vi "DFD Probe Check Filter Bank.vi"(1 "filter bank in":T1={"mFBank_AnalysisFilters"=[], "mFBank_SynthesisFilters"=[], "mFBank_#Bands"=0, "mFBank_ProcMethod"=enum."General", "mFBank_Coeffs"=[], "mFBank_Gain"=1.0, "mFBank_Delay"=0, "mFBank_Type"=0} {"mFBank_SynthesisFilters"."mMRate_SumWl" min=1 max=32 step=1; "mFBank_SynthesisFilters"."mMRate_InputIwl" min=1 max=32 step=1; "mFBank_SynthesisFilters"."mMRate_GainWl" min=1 max=32 step=1; "mFBank_SynthesisFilters"."mMRate_OutputWl" min=1 max=32 step=1; "mFBank_SynthesisFilters"."mMRate_InputWl" min=1 max=32 step=1; "mFBank_SynthesisFilters"."mMRate_CoefWl" min=1 max=32 step=1; "mFBank_SynthesisFilters"."mMRate_Mode" items=["Default"=-1, "No Rate Change"=0, "Interpolation"=1, "Decimation"=2, "Interpolated"=3, "Rational"=4]; "mFBank_AnalysisFilters"."mMRate_SumWl" min=1 max=32 step=1; "mFBank_AnalysisFilters"."mMRate_InputIwl" min=1 max=32 step=1; "mFBank_AnalysisFilters"."mMRate_GainWl" min=1 max=32 step=1; "mFBank_AnalysisFilters"."mMRate_OutputWl" min=1 max=32 step=1; "mFBank_AnalysisFilters"."mMRate_InputWl" min=1 max=32 step=1; "mFBank_AnalysisFilters"."mMRate_CoefWl" min=1 max=32 step=1; "mFBank_AnalysisFilters"."mMRate_Mode" items=["Default"=-1, "No Rate Change"=0, "Interpolation"=1, "Decimation"=2, "Interpolated"=3, "Rational"=4]; "mFBank_Type" items=["Uniform", "Non-Uniform"]}) -> (0 "Boolean":bool)   [LabVIEW 2017, in "NI_DigFilterLicensed.lvlib"]
uses:
  <vilib>/addons/Digital Filter Design/NI_DigFilterLicensed.lvlib
  <vilib>/addons/Digital Filter Design/FilterBank.llb/Object/DFD Filter Bank Obj.ctl
  <vilib>/addons/Digital Filter Design/_Objects.llb/DFD Multirate Filter Obj.ctl
  <vilib>/addons/Digital Filter Design/_Objects.llb/DFD Multirate Mode.ctl
  <vilib>/addons/Digital Filter Design/_Objects.llb/DFD Coef Norm Type.ctl
  <vilib>/addons/Digital Filter Design/_Objects.llb/DFD Round-off Mode.ctl
  <vilib>/addons/Digital Filter Design/_Objects.llb/DFD FXP MRate Multiply Mode.ctl
  <vilib>/addons/Digital Filter Design/FilterBank.llb/Object/DFD Filter Bank Processing Method.ctl
  <vilib>/addons/Digital Filter Design/FilterBank.llb/Object/DFD Filter Bank Type.ctl
  <vilib>/addons/Digital Filter Design/NI_DigFilter_FilterBank.lvlib
panel:
  in  "Tab Control":T9(tab)
  in  "order":i32=-1 caption="Filter bank order" min=2
  in  "#bands":i32 caption="Number of bands" min=1 max=1 step=1
  in  "dist_in dB":bool=TRUE caption="Magnitude in dB"
  out "Mag distortion":cluster{dbl[], "values":dbl[]}(graph)
  in  "resp_in dB":bool=TRUE caption="Magnitude in dB"
  out "Mag responses":cluster{"Y":dbl[], "Y":dbl[]}[](graph)
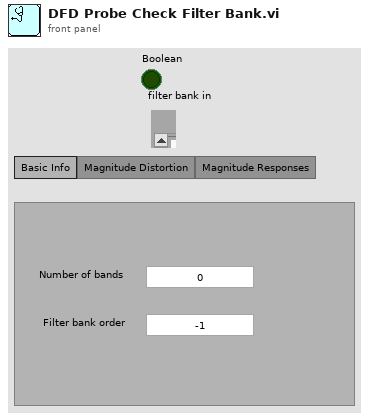
[diagram p1: front panel]
types:
  T1 = typedef "NI_DigFilter_FilterBank.lvlib/DFD Filter Bank Obj.ctl" = cluster{"mFBank_AnalysisFilters":T2[], "mFBank_SynthesisFilters":T2[], "mFBank_#Bands":i32, "mFBank_ProcMethod":T7, "mFBank_Coeffs":dbl[], "mFBank_Gain":dbl, "mFBank_Delay":i32, "mFBank_Type":T8}
  T2 = typedef "NI_DigFilterLicensed.lvlib/DFD Multirate Filter Obj.ctl" = cluster{"mMRate_Structure":enum16{"CIC", "FIR", "IIR", "Lattice"}, "mMRate_Mode":T3, "mMRate_Factor":i32, "mMRate_FIRParams":cluster{"mMRate_FIR_H":dbl[], "mMRate_FIR_IsNyquist?":bool, "mMRate_FIR_IsSymmetric?":bool}, "mMRate_CICParams":cluster{"mMRate_CIC_#Stage":i32, "mMRate_CIC_Lag":i32, "mMRate_CIC_Type":enum16{"Lowpass", "Highpass"}}, "mMRate_Order":i32, "mMRate_Version":string, "mMRate_Comments":string, "mMRate_RationalFactor":cluster{"mMRate_L":i32, "mMRate_M":i32}, "mMRate_Fs":dbl, "mMRate_Quantized?":bool, "mMRate_QFilterGain":dbl, "mMRate_CoefWl":i16, "mMRate_Scaling":cluster{"mMRate_ScaleByPowerOf2?":bool, "mMRate_ScaleType":T4}, "mMRate_InputWl":i16, "mMRate_OutputWl":i16, "mMRate_OutputMode":T5, "mMRate_MultMode":T6, "mMRate_BitPruning":bool, "mMRate_GainWl":i16, "mMRate_OutputFwl":i16, "mMRate_SumIwl":i16, "mMRate_InputIwl ":i16, "mMRate_SumWl":i16, "mMRate_CoefIwl":i16}
  T3 = typedef "NI_DigFilterLicensed.lvlib/DFD Multirate Mode.ctl" = i16
  T4 = typedef "NI_DigFilterLicensed.lvlib/DFD Coef Norm Type.ctl" = enum16{"No Norm", "Time Domain 1-Norm", "Time Domain 2-Norm", "Time Domain Inf-Norm"}
  T5 = typedef "NI_DigFilterLicensed.lvlib/DFD Round-off Mode.ctl" = enum16{"Nearest", "Truncation"}
  T6 = typedef "NI_DigFilterLicensed.lvlib/DFD FXP MRate Multiply Mode.ctl" = enum16{"Truncated", "Full"}
  T7 = typedef "NI_DigFilter_FilterBank.lvlib/DFD Filter Bank Processing Method.ctl" = enum16{"General", "2-Band QMF Lattice", "Cosine-Modulated"}
  T8 = typedef "NI_DigFilter_FilterBank.lvlib/DFD Filter Bank Type.ctl" = u16
  T9 = enum32{"Basic Info", "Magnitude Distortion", "Magnitude Responses"}
  T10 = enum8{"Enabled", "Disabled", "Disabled and Grayed Out"}
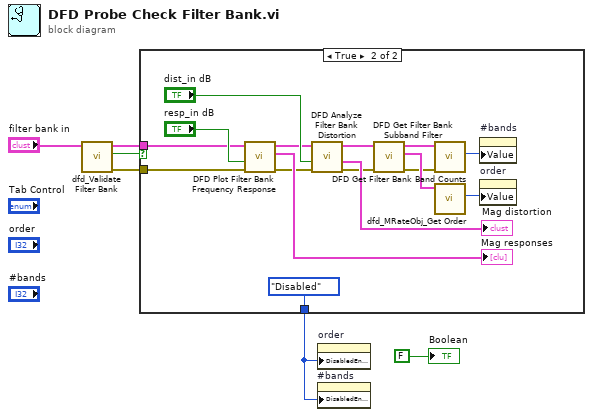
[diagram p0: block diagram]
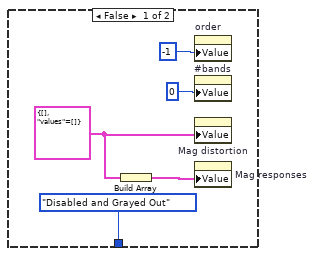
[diagram p2: hidden frame]
diagram:
  n1 = call <vilib>:"dfd_Validate Filter Bank.vi"("filter banks in"="filter bank in") -> ("error out"=w3:errorcluster, "is Valid?"=w4:bool, "filter bank out"=w5:T1)  [unwired: 8 in]
  n2 = case shown="True" w4 {
    tunnel: w5 -> [_ w16]
    tunnel: w3 -> [_ w15]
    tunnel: [T10."Disabled and Grayed Out" ("Disabled") T10."Disabled" ("Disabled")] -> w1
    frame False {
      w9 = cluster{dbl[], "values":dbl[]} {[], "values"=[]} ("Mag distortion")
      n3 = Build Array(w9) -> (w10:cluster{dbl[], "values":dbl[]}[])
      n4 = property on="order" class="DigNum (strict)"("Value"=-1 ("order")) -> ()  [unwired: 2 in, 2 out]
      n5 = property on="#bands" class="DigNum (strict)"("Value"=0 ("#bands")) -> ()  [unwired: 2 in, 2 out]
      n6 = property on="Mag distortion" class="XYGraph (strict)"("Value"=w9) -> ()  [unwired: 2 in, 2 out]
      n7 = property on="Mag responses" class="XYGraph (strict)"("Value"=w10) -> ()  [unwired: 2 in, 2 out]
    }
    frame True {
      n8 = call <vilib>:"DFD Plot Filter Bank Frequency Response.vi"("error in (no error)"=w15, "dB on? (T)"="resp_in dB", "filter bank in"=w16) -> ("error out"=w18:errorcluster, "magnitude responses"=→"Mag responses":cluster{"Y":dbl[], "Y":dbl[]}[], "filter bank out"=w17:T1)  [unwired: 5 in, 1 out]
      n9 = call <vilib>:"DFD Analyze Filter Bank Distortion.vi"("error in (no error)"=w18, "dB on? (T)"="dist_in dB", "filter bank in"=w17) -> ("error out"=w20:errorcluster, "magnitude distortion"=→"Mag distortion":cluster{dbl[], "values":dbl[]}, "filter bank out"=w19:T1)  [unwired: 4 in, 2 out]
      n10 = call <vilib>:"DFD Get Filter Bank Subband Filter.vi"("error in (no error)"=w20, "filter bank in"=w19) -> ("error out"=w13:errorcluster, "subband filter"=w22:T2, "filter bank out"=w14:T1)  [unwired: 7 in]
      n11 = call <vilib>:"DFD Get Filter Bank Band Counts.vi"("error in (no error)"=w13, "filter bank in"=w14) -> ("band counts"=w12:i32)  [unwired: 7 in, 2 out]
      n12 = call <vilib>:"dfd_MRateObj_Get Order.vi"("multirate filter in"=w22) -> ("order"=w21:i32)  [unwired: 9 in, 1 out]
      n13 = property on="#bands" class="DigNum (strict)"("Value"=w12) -> ()  [unwired: 2 in, 2 out]
      n14 = property on="order" class="DigNum (strict)"("Value"=w21) -> ()  [unwired: 2 in, 2 out]
    }
  }
  n15 = property on="order" class="DigNum (strict)"("DisabledEnum"=w1) -> ()  [unwired: 2 in, 2 out]
  n16 = property on="#bands" class="DigNum (strict)"("DisabledEnum"=w1) -> ()  [unwired: 2 in, 2 out]
  "Boolean" <- FALSE ("Boolean")
